vi "Move Window.vi"(4 "error in (no error)":errorcluster, 5 "new position (0,0)":cluster{"left":i16, "top":i16}, 6 "window name (\"\")":string, 7 "window refnum (NaWR)":T1) -> (0 "error out":errorcluster, 1 "prev position":cluster{"left":i16, "top":i16}, 3 "window refnum out":T1)   [LabVIEW 2023, in "WINUTIL.lvlib"]
doc: "This function will move the window named in the 'window name' input or identified by the 'window refnum' from its present location to that defined in the 'new position' cluster. Coordinates are pixels relative to upper left corner of the screen.\n\nIf the function is successful, then:\n'window refnum out' = 'window refnum' if window refnum in is valid;\n'window refnum out' is a new window refnum if 'window refnum' is not valid and 'window name' a valid name for a window.\n\nIf the window cannot be found, an error will be returned and window refnum out will be 'Not a Valid Window RefNum'."
uses:
  WINUTIL.lvlib
  Window Refnum.ctl
  user32.dll
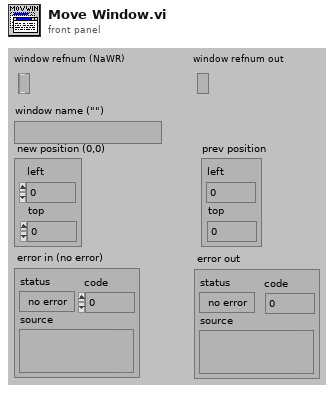
[diagram p1: front panel]
types:
  T1 = typedef "WINUTIL.lvlib/Window Refnum.ctl" = refnum<k1>
  T2 = typedef "WINUTIL.lvlib/Window Rectangle.ctl" = cluster{"left":i16, "top":i16, "right":i16, "bottom":i16}
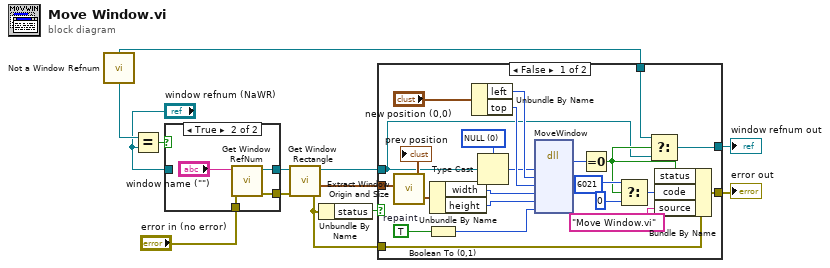
[diagram p0: block diagram]
diagram:
  n1 = call "Not a Window Refnum.vi"() -> ("Not a Window Refnum"=w3:T1)
  n2 = Equal?(x=w3, y="window refnum (NaWR)") -> (x = y?=w4:bool)
  n3 = case shown="True" w4 {
    tunnel: "error in (no error)" -> [w14 w17]
    tunnel: [w14 w15] -> w10
    tunnel: [w13 w16] -> w7
    tunnel: "window refnum (NaWR)" -> [w13 _]
    frame False {
    }
    frame True {
      n4 = call "Get Window RefNum.vi"("error in (no error)"=w17, "window name (\"\")"="window name (\"\")") -> ("error out"=w15:errorcluster, "window refnum (NaWR)"=w16:T1)  [unwired: 6 out]
    }
  }
  n5 = call "Get Window Rectangle.vi"("error in (no error)"=w10, "window refnum (NaWR)"=w7) -> ("error out"=w5:errorcluster, "window rect"=w6:T2, "window refnum out"=w8:T1)  [unwired: 1 in, 2 out]
  n6 = Unbundle By Name(w5) -> ("status"=w12:bool)
  n7 = case shown="False" w12 {
    tunnel: w6 -> [w29 _]
    tunnel: [w27 w43] -> w11
    tunnel: w8 -> [w19 w42]
    tunnel: w5 -> [w28 w43]
    tunnel: w3 -> [w20 _]
    tunnel: [w23 w42] -> w2
    frame False {
      w21 = u32 0 items=["NULL"]
      w37 = TRUE  # repaint
      n8 = call "Extract Window Origin and Size.vi"("window rect"=w29) -> ("window origin"=→"prev position":cluster{"left":i16, "top":i16}, "window size"=w38:cluster{"width":i16, "height":i16})
      n9 = Boolean To (0,1)(Boolean=w37) -> (0, 1=w36:i16)
      n10 = Unbundle By Name(w38) -> ("width"=w35:i16, "height"=w34:i16)
      n11 = Unbundle By Name("new position (0,0)") -> ("left"=w40:i16, "top"=w39:i16)
      n12 = Type Cast(type=w21, x=w19) -> (*(type *) &x=w22:u32)
      n13 = dll-call lib="USER32.DLL" fn="MoveWindow"("hWnd"=w22, "left"=w40, "top"=w39, "right"=w35, "bottom"=w34, "repaint"=w36) -> ("error"=w33:i32)  [unwired: 4 in, 7 out]
      n14 = Equal To 0?(x=w33) -> (x = 0?=w24:bool)
      n15 = Select(t=6021, s=w24, f=0) -> (s? t:f=w25:i32)
      n16 = Select(t=w20, s=w24, f=w19) -> (s? t:f=w23:T1)
      n17 = Bundle By Name(cluster=w28, "status"=w24, "code"=w25, "source"="Move Window.vi") -> (w27:errorcluster)
    }
    frame True {
    }
  }
  "error out" <- w11
  "window refnum out" <- w2
